vi "Set Tx Generic File Path.vi"(8 "error in":errorcluster, 10 "frame array file path":path, 11 "custom device ref in":T1 format="%.0x") -> (0 "error out":errorcluster, 3 "custom device ref out out":T1 format="%.0x")   [LabVIEW 2020, in "AIM ARINC 664 Scripting.lvlib"]
uses:
  AIM ARINC 664 Scripting.lvlib
  <vilib>/NI VeriStand/Custom Device API/Custom Device Item Ref.ctl
  Constants.vi
  <vilib>/NI VeriStand/Custom Device Tools/Custom Device Utility Library/NI VeriStand - Search for Item by GUID.vi
  <vilib>/NI VeriStand/Custom Device API/Set Item Property (Dependent File).vi
  <vilib>/NI VeriStand/Custom Device API/Custom Device API.lvlib
  <vilib>/NI VeriStand/Custom Device Tools/Custom Device Utility Library/Custom Device Utility Library.lvlib
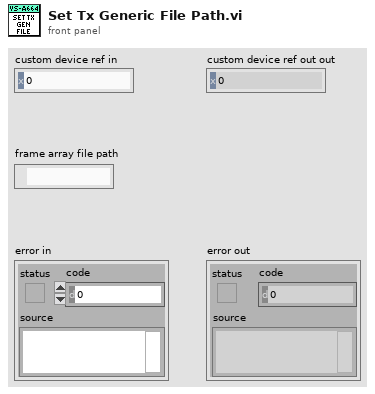
[diagram p1: front panel]
types:
  T1 = typedef "Custom Device API.lvlib/Custom Device Item Ref.ctl" = u64
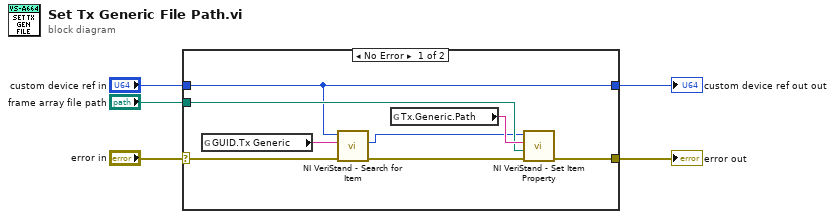
[diagram p0: block diagram]
diagram:
  n1 = case shown="No Error" "error in" {
    selector: "error in" -> [w11 w15]
    tunnel: "custom device ref in" -> [w8 w14]
    tunnel: [w13 w15] -> w4
    tunnel: [w8 w14] -> w3
    tunnel: "frame array file path" -> [w10 _]
    frame No Error {
      n2 = global read "Constants.vi" "GUID.Tx Generic"() -> (w6:string)
      n3 = call-poly <vilib>:"NI VeriStand - Search for Item.vi"("error in"=w11, "Item GUID"=w6, "Section Ref in"=w8) -> ("error out"=w9:errorcluster, "Item Ref"=w7:T1)  [unwired: 5 in, 2 out]
      n4 = global read "Constants.vi" "Tx.Generic.Path"() -> (w12:string)
      n5 = call-poly <vilib>:"NI VeriStand - Set Item Property.vi"("error in (no error)"=w9, "Path"=w10, "Property Name"=w12, "Item Ref in"=w7) -> ("error out"=w13:errorcluster)  [unwired: 5 in, 2 out]
    }
    frame Error {
    }
  }
  "error out" <- w4
  "custom device ref out out" <- w3
